vi "Send Update Elevator Location.vi"(7 "Message Priority (Normal)":T2=enum."Normal", 8 "error in (no error)":errorcluster, 10 "Elevator Location":T1, 11 "Message Enqueuer":refnum<class "Message Enqueuer.lvclass">) -> (0 "error out":errorcluster, 3 "Message Enqueuer out":refnum<class "Message Enqueuer.lvclass">)   [LabVIEW 2022 SP3, in "Sim Display Console Actor.lvlib" / "Update Elevator Location Msg.lvclass"]
doc: "This VI sends the message to an actor."
uses:
  Update Elevator Location Msg.lvclass
  <vilib>/ActorFramework/Message Enqueuer/Message Enqueuer.lvclass
  <vilib>/ActorFramework/Message Enqueuer/Message Priority.ctl
  Elevator Controller Actor/Floor -Enum.ctl
  C:/Program Files/National Instruments/LabVIEW 2022/vi.lib/ActorFramework/Message/Message.lvclass
  Update Elevator Location Msg.lvclass/Update Elevator Location Msg.ctl
  <vilib>/ActorFramework/Message Enqueuer/Message Enqueuer.lvclass/Message Enqueuer.ctl
  <vilib>/ActorFramework/Message Priority Queue/Priority Enqueue.vi
  C:/Workspace/CLA/Elevator AF_2022_2nd/Sim Display Console Actor/Sim Display Console Actor Messages/Update Elevator Location Msg/Update Elevator Location Msg.lvclass
  Elevator Controller Actor/Sim Display Console Actor.lvclass
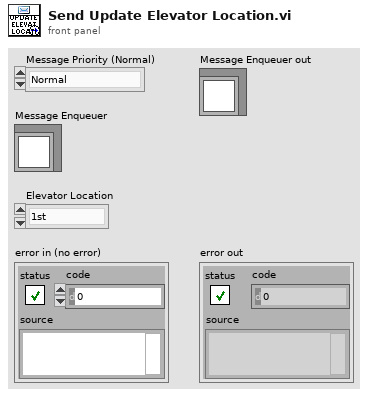
[diagram p1: front panel]
types:
  T1 = typedef "Sim Display Console Actor.lvlib/Sim Display Console Actor.lvclass/Floor -Enum.ctl" = enum16{"1st", "2nd", "3rd", "4th"}
  T2 = typedef "Actor Framework.lvlib/Message Enqueuer.lvclass/Message Priority.ctl" = enum16{"Low", "Normal", "High"}
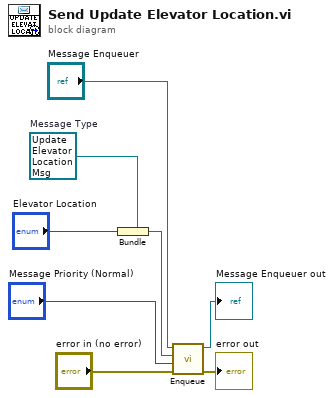
[diagram p0: block diagram]
diagram:
  w5 = refnum<class "Update Elevator Location Msg.lvclass"> refnum  # Message Type
  n1 = Bundle(cluster=w5, "Elevator Location") -> (w4:refnum<class "Update Elevator Location Msg.lvclass">)
  n2 = call <vilib>:"Enqueue.vi"("error in (no error)"="error in (no error)", "Message Priority (Normal)"="Message Priority (Normal)", "Message"=w4, "Message Enqueuer in"="Message Enqueuer") -> ("error out"=→"error out":errorcluster, "Message Enqueuer in"=→"Message Enqueuer out":refnum<class "Message Enqueuer.lvclass">)  [unwired: 6 in]
